vi "Get SQL formatted value.vi"(8 "error in (no error)":errorcluster, 11 "Column in":refnum<class "Composed Column.lvclass">) -> (0 "error out":errorcluster, 2 "Formatted Value":string, 3 "Column out":refnum<class "Composed Column.lvclass">)   [LabVIEW 2020, in "Composed Columns.lvlib" / "Composed Column.lvclass"]
uses:
  Composed Column.lvclass
  Composed Column.lvclass/Composed Column.ctl
  Value Type/Value Type.lvclass
  Composed Columns/Value Source Interface Class/Value Source.lvclass
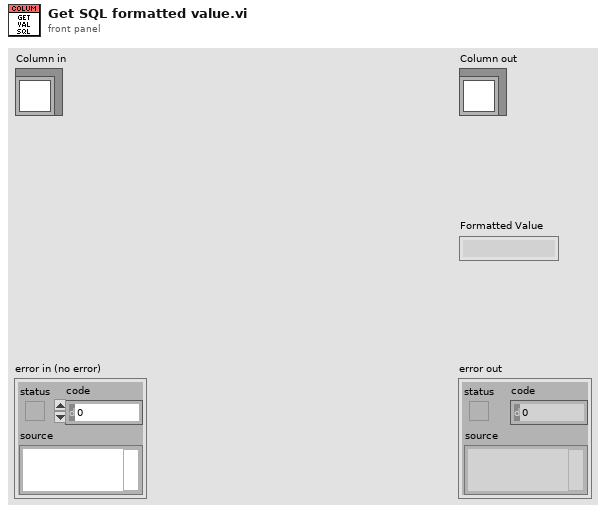
[diagram p1: front panel]
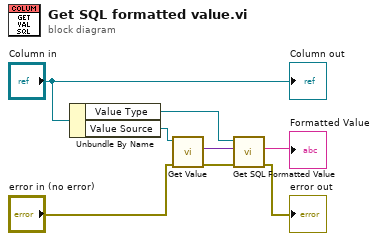
[diagram p0: block diagram]
diagram:
  n1 = Unbundle By Name("Column in") -> ("Value Type"=w5:refnum<class "Value Type.lvclass">, "Value Source"=w4:refnum<class "Value Source.lvclass">)
  n2 = call-dynamic "Get Value.vi"("error in (no error)"="error in (no error)", "Value Source in"=w4) -> ("error out"=w2:errorcluster, "Value"=w6:variant)  [unwired: 7 in, 1 out]
  n3 = call-dynamic "Get SQL Formatted Value.vi"("error in (no error)"=w2, "Value"=w6, "Value Type in"=w5) -> ("error out"=→"error out":errorcluster, "SQL Formatted Value"=→"Formatted Value":string)  [unwired: 6 in, 1 out]
  "Column out" <- "Column in"
